vi "Set Fill Mode.vi"(8 "error in (no error)":errorcluster, 10 "Fill Mode":T1="ON", 11 "Instrument.1820 in":refnum<class "Instrument.Oxford1820.lvclass">) -> (0 "error out":errorcluster, 2 "Response":string, 3 "Instrument.1820 in":refnum<class "Instrument.Oxford1820.lvclass">)   [LabVIEW 2019, in "Instrument.Oxford1820.lvclass"]
uses:
  Instrument.Oxford1820.lvclass
  Typedefs/Fill Mode-Combo.ctl
  Typedefs/Instrument.Oxford1820.protectedCommands-enum.ctl
  55508935-8232-4deb-842d-8d1c18a8b24e.vi/722a0f26-baea-410a-9d3f-4622907dceeb.vi
  55508935-8232-4deb-842d-8d1c18a8b24e.vi/41f0bcce-007e-4fad-99b1-182ca59d5085.vi
  <vilib>/Utility/Data Type/Get Type Information.vi
  <vilib>/JDP Science/JSONtext/JSON text to Variant.vi
  <vilib>/JDP Science/JSONtext/LVClass Serializer/JSONtext LVClass Serializer.lvclass
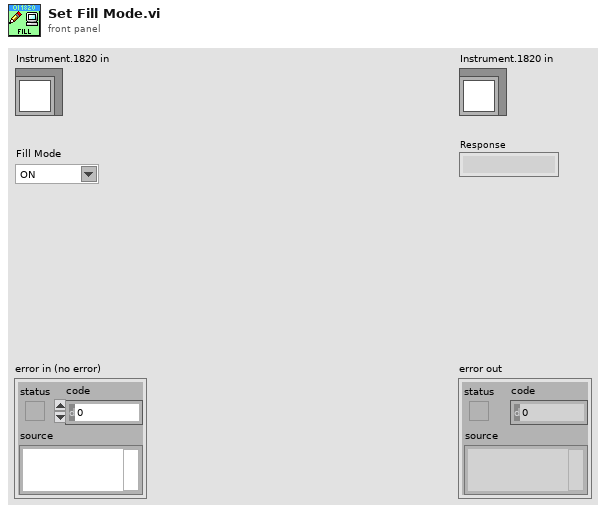
[diagram p1: front panel]
types:
  T1 = typedef "Instrument.Oxford1820.lvclass/Fill Mode-Combo.ctl" = string
  T2 = typedef "Instrument.Oxford1820.lvclass/Instrument.Oxford1820.protectedCommands-enum.ctl" = enum16{"Hold", "RampToSet", "RampToZero", "Clamp", "setTarget", "setSwitchHeat", "setLambda", "setFillMode", "setNeedleValve", "getStatus", "getTarget", "getSwitchHeat", "getPSUField", "setSequenceStatus"}
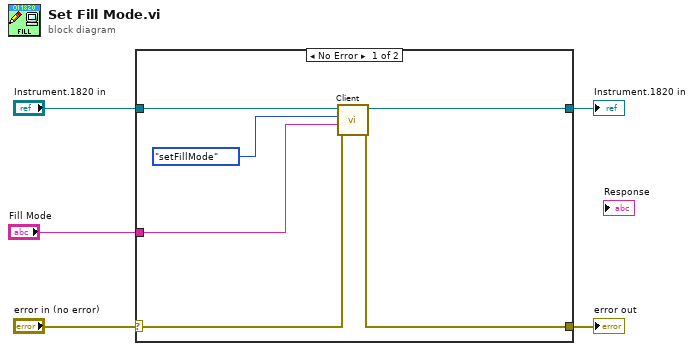
[diagram p0: block diagram]
diagram:
  n1 = case shown="No Error" "error in (no error)" {
    selector: "error in (no error)" -> [w8 w13]
    tunnel: [w7 w13] -> w4
    tunnel: [w6 w12] -> w2
    tunnel: "Instrument.1820 in" -> [w11 w12]
    tunnel: "Fill Mode" -> [w9 _]
    frame No Error {
      n2 = call-dynamic "Client.vi"("error in (no error)"=w8, "Data in"=w9, "Command in"=Instrument.Oxford1820.protectedCommands-enum."setFillMode" ("Commands"), "Instrument in"=w11) -> ("error out"=w7:errorcluster, "Instrument out"=w6:refnum<class "Instrument.Oxford1820.lvclass">)  [unwired: 4 in, 2 out]
    }
    frame Error {
    }
  }
  "error out" <- w4
  "Instrument.1820 in" <- w2
